vi "Start Call.vi"   [LabVIEW 2024, in "serenial.io-ase.lvlib" / "ase.lvclass"]
doc: "<B>Start an Asynchronous System Executable Call</B>\n\nThe executable should either be specified as a name available in this process's PATH variable using the \"command\" polymorphic VI instance or the absolute path to the executable can be used with the \"exe-args\" polymorphic instance. These instances reflect the two options the underlying boost library uses to create a child process. See https://www.boost.org/doc/libs/1_77_0/doc/html/boost_process/design.html#boost_process.design.arg_cmd_style for more information.\n\nThe User Events References to generate \"Standard Output\", \"Standard Error\" and \"Did Exit\" events can be supplied or omitted as required. <B>Ensure that the event registration process for any User Events passed to this VI has already been undertaken</B>.\n\nThe configuration class allows for override of certain behaviours such as the regular expression used to match the breaks in the Standard Out and Standard Error to be specified.\n\nThis VI generates the following errors:\n-4601: Poorly formatted/incorrect Regular Expression supplied.\n-5691000: Internal Library Error. <Check Error Message for more details>\n-5691301: Unable to launch the executable. <Check Error Message for more details>\n-5691305: Executable name/path parameter cannot be an empty value."
uses:
  ase.lvclass
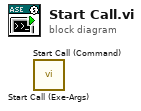
[diagram p0: block diagram]
diagram:
  n1 = call "Start Call (Exe-Args).vi"() -> ()  [unwired: 10 in, 2 out]
  n2 = call "Start Call (Command).vi"() -> ()  [unwired: 10 in, 2 out]
